vi "Close Dynamic Dialog.vi"(8 "error in (no error)":errorcluster, 10 "Close? [T]":bool=TRUE) -> (0 "error out":errorcluster)   [LabVIEW 2020, in "Multiple Errors.lvclass"]
uses:
  Multiple Errors.lvclass
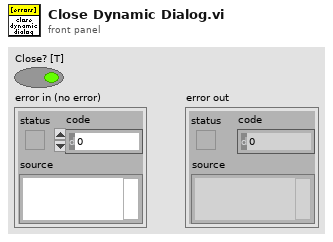
[diagram p1: front panel]
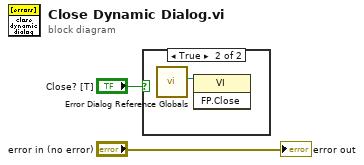
[diagram p0: block diagram]
diagram:
  n1 = case shown="True" "Close? [T]" {
    frame False {
    }
    frame True {
      n2 = call "Error Dialog Reference Globals.vi"() -> ("VI reference"=w3:refnum<vi>)  [unwired: 10 in, 1 out]
      n3 = invoke class="VI" method="FP.Close"(reference=w3) -> ()  [unwired: 2 in, 3 out]
    }
  }
  "error out" <- "error in (no error)"
